vi "Get RPTID Data.vi"(8 "error in (no error)":errorcluster, 11 "RPTID":u32) -> (0 "error out":errorcluster, 2 "OK":bool, 3 "Value":cluster{"Format Code":T1, "Value":variant}[](array[cluster]))   [LabVIEW 2020, in "SECS Scenarios.lvlib" / "09-Host Requsts Individual Report.lvclass"]
uses:
  09-Host Requsts Individual Report.lvclass
  SECS Communication/SECS-II Class/Format Code.ctl
  SECS Communication/SECS Data Class/Get SVID Data.vi
  SECS Communication/SECS Data Class/Get ECID Data.vi
  SECS Communication/SECS Data Class/Get ALID Data.vi
  09-Host Requsts Individual Report.lvclass/09-Host Requsts Individual Report.ctl
  SECS Communication/SECS Data Class/SECS Data Class.lvclass
  SECS Communication/SECS-II Class/SECS-II Class.lvclass
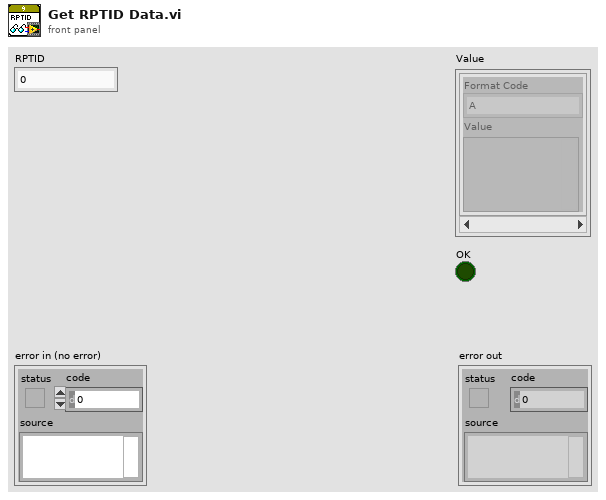
[diagram p1: front panel]
types:
  T1 = typedef "SECS Communication.lvlib/SECS-II Class.lvclass/Format Code.ctl" = enum16{"L", "A", "B", "Boolean", "J", "I1", "I2", "I4", "I8", "U1", "U2", "U4", "U8", "F4", "F8", "Char"}
  T2 = typedef "SECS Communication.lvlib/SECS Data Class.lvclass/RPTID Data.ctl" = cluster{"RPTID":u32, "Report Information":string[], "Dynamic":bool}
  T3 = typedef "SECS Communication.lvlib/SECS Data Class.lvclass/SVID Data.ctl" = cluster{"SVID":u32, "Name":string, "Description":string, "Format Code":T1, "Unit":string, "Source":string, "Data":variant}
  T4 = typedef "SECS Communication.lvlib/SECS Data Class.lvclass/ECID Data.ctl" = cluster{"ECID":u32, "Name":string, "Description":string, "Format Code":T1, "Unit":string, "Max":dbl, "Min":dbl, "Default":string, "Source":string, "Data":variant}
  T5 = typedef "SECS Communication.lvlib/SECS Data Class.lvclass/ALID Data.ctl" = cluster{"Enable":bool, "ALID":u32, "Name":string, "Description":string, "Source":string, "Status":enum16{"Null", "Normal", "Abnormal", "Warning"}}
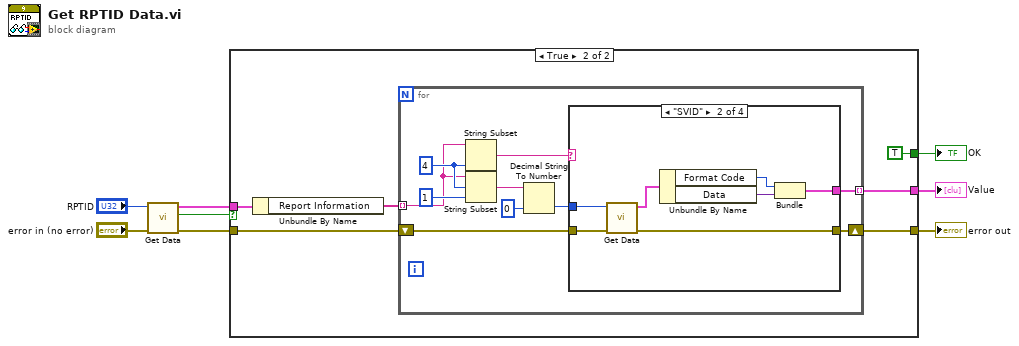
[diagram p0: block diagram]
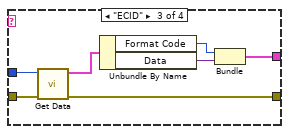
[diagram p4: hidden frame]
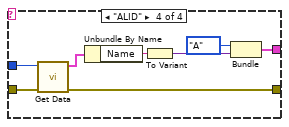
[diagram p5: hidden frame]
diagram:
  n1 = call-poly "Get Data.vi"("error in"="error in (no error)", "RPTID"="RPTID") -> ("error out"=w5:errorcluster, "Find?"=w4:bool, "RPTID Data"=w7:T2)  [unwired: 7 in]
  n2 = case shown="True" w4 {
    tunnel: w7 -> [_ w15]
    tunnel: w5 -> [w9 w14]
    tunnel: [w9 w12] -> w3
    tunnel: [_ w11] -> w2
    tunnel: [_ TRUE] -> w1
    frame False {
    }
    frame True {
      n3 = Unbundle By Name(w15) -> ("Report Information"=w13:string[])
      n4 = for {
        shift-right: [w17] -> w12
        shift-left: w14 -> [w19]
        tunnel: w13 -> [w16] mode=indexing
        tunnel: [w18] -> w11 mode=indexing
        w25 = 4 ("length (rest)")
        n5 = String Subset(string=w16, length (rest)=w25) -> (substring=w21:string)  [unwired: 1 in]
        n6 = String Subset(string=w16, offset (0)=w25, length (rest)=1 ("length (rest)")) -> (substring=w23:string)
        n7 = Decimal String To Number(string=w23, default (0L)=u32 0 ("default (0 I32)")) -> (number=w20:u32)  [unwired: 1 in, 1 out]
        n8 = case shown="\"SVID\"" w21 {
          tunnel: w20 -> [_ w32 w39 w44]
          tunnel: w19 -> [w26 w33 w40 w45]
          tunnel: [_ w28 w35 w48] -> w18
          tunnel: [w26 w27 w34 w43] -> w17
          frame Default {
          }
          frame "SVID" {
            n9 = call-poly "Get Data.vi"("error in"=w33, "SVID"=w32) -> ("error out"=w27:errorcluster, "SVID Data"=w31:T3)  [unwired: 7 in, 1 out]
            n10 = Unbundle By Name(w31) -> ("Format Code"=w29:T1, "Data"=w30:variant)
            n11 = Bundle("Format Code"=w29, "Data"=w30) -> (w28:cluster{"Format Code":T1, "Data":variant})  [unwired: 1 in]
          }
          frame "ECID" {
            n12 = call-poly "Get Data.vi"("error in"=w40, "ECID"=w39) -> ("error out"=w34:errorcluster, "ECID Data"=w38:T4)  [unwired: 7 in, 1 out]
            n13 = Unbundle By Name(w38) -> ("Format Code"=w36:T1, "Data"=w37:variant)
            n14 = Bundle("Format Code"=w36, "Data"=w37) -> (w35:cluster{"Format Code":T1, "Data":variant})  [unwired: 1 in]
          }
          frame "ALID" {
            n15 = call-poly "Get Data.vi"("error in"=w45, "ALID"=w44) -> ("error out"=w43:errorcluster, "ALID Data"=w42:T5)  [unwired: 7 in, 1 out]
            n16 = Unbundle By Name(w42) -> ("Name"=w41:string)
            n17 = To Variant(anything=w41) -> (Variant=w46:variant)
            n18 = Bundle("Format Code"=Format_Code."A", "Variant"=w46) -> (w48:cluster{"Format Code":T1, "Variant":variant})  [unwired: 1 in]
          }
        }
      }
    }
  }
  "error out" <- w3
  "Value" <- w2
  "OK" <- w1
